vi "swapBits.vi"(10 "In":u8 format="%b") -> (2 "Out":u8 format="%b")   [LabVIEW 2013]
panel:
  out "Boolean array":bool[](array[boolean])
  in  "stop":bool
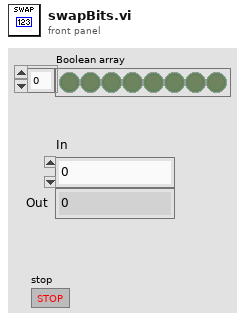
[diagram p1: front panel]
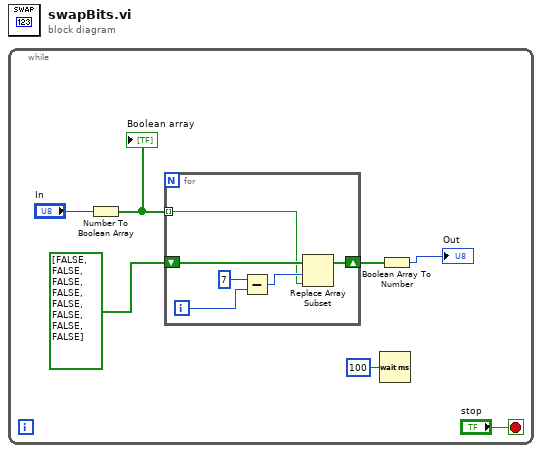
[diagram p0: block diagram]
diagram:
  n1 = while {
    stop <- "stop" stop-if-true
    n2 = Number To Boolean Array(number="In") -> (Boolean array=w5:bool[])
    "Boolean array" <- w5
    n3 = for {
      tunnel: w5 -> [w8] mode=indexing
      shift-right: [w9] -> w3
      shift-left: bool[] [FALSE, FALSE, FALSE, FALSE, FALSE, FALSE, FALSE, FALSE] -> [w13]
      i -> [w11]
      n4 = Subtract(x=7, y=w11) -> (x-y=w12:i32)
      n5 = Replace Array Subset(array=w13, new element=w8, index=w12) -> (w9:bool[])
    }
    n6 = Wait (ms)(milliseconds to wait=u32 100) -> ()  [unwired: 1 out]
    n7 = Boolean Array To Number(Boolean array=w3) -> (number=→"Out":u32)
  }
